vi "Z900_navX_Util_EncodeProtocol_UnsignedThousandths.vi"(1 "Unsigned Thousandths (0.000)":dbl[](array[numeric])) -> (0 "Little Endian":u8[](array[numeric]))   [LabVIEW 2015, in "navX Library v2.lvlib"]
uses:
  navX Library v2.lvlib
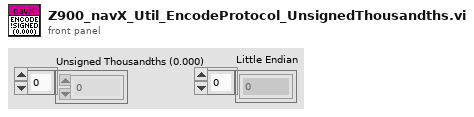
[diagram p1: front panel]
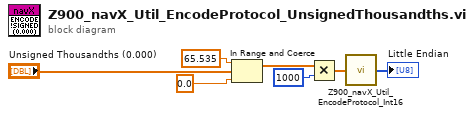
[diagram p0: block diagram]
diagram:
  n1 = In Range and Coerce(upper limit=65.535, x="Unsigned Thousandths (0.000)", lower limit=0.0) -> (coerced(x)=w4:dbl[])  [unwired: 1 out]
  n2 = Multiply(x=w4, y=1000) -> (x*y=w6:dbl[])
  n3 = call "Z900_navX_Util_EncodeProtocol_Int16.vi"("Int16"=w6) -> ("Little Endian"=→"Little Endian":u8[])
